vi "JoystickDeadBand.vi"(11 "JoystickInput":dbl) -> (3 "JoystickAfterDeadband":dbl)   [LabVIEW 2017]
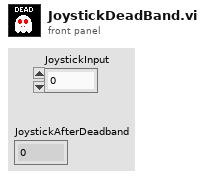
[diagram p1: front panel]
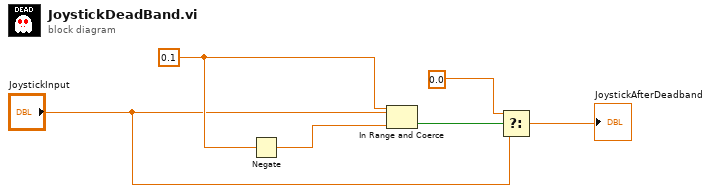
[diagram p0: block diagram]
diagram:
  w5 = 0.1 ("x")
  n1 = Negate(x=w5) -> (-x=w6:dbl)
  n2 = In Range and Coerce(upper limit=w5, x="JoystickInput", lower limit=w6) -> (In Range?=w3:bool)  [unwired: 1 out]
  n3 = Select(t=0.0, s=w3, f="JoystickInput") -> (s? t:f=→"JoystickAfterDeadband":dbl)
